vi "Configure.vi"(6 "CMD Prefix":string, 7 "CMDs":string[](array[string]), 8 "error in":errorcluster, 9 "JSON Settings Path":string, 10 "JSON Keys":string[](array[string]), 11 "Continuous Waveform Acq CFG in":refnum<class "Continuous Waveform Acq CFG.lvclass">) -> (0 "error out":errorcluster, 3 "Continuous Waveform Acq CFG out":refnum<class "Continuous Waveform Acq CFG.lvclass">)   [LabVIEW 2023, in "Continuous Waveform Acq CFG.lvclass"]
uses:
  Continuous Waveform Acq CFG.lvclass
  E:/git/HAL/Configuration Base/Configuration Base.lvclass
  E:/git/HAL/Scope VISA/Configuration/Scope VISA CFG.lvclass
  HAL/Scope VISA/Configuration/Scope VISA CFG.lvclass/Scope VISA CFG.ctl
  HAL/Configuration Base/Configuration Base.lvclass/Configuration Base.ctl
  <vilib>/JDP Science/JSONtext/Next JSON Value.vi
  <vilib>/JDP Science/JSONtext/String Subset.vi
  <vilib>/JDP Science/JSONtext/Parsing/Advance past next JSON Value (inlined COPY).vi
  <vilib>/JDP Science/JSONtext/Parsing/Advance past whitespace.vi
  <vilib>/JDP Science/JSONtext/Parsing/Advance past String.vi
  <vilib>/JDP Science/JSONtext/Parsing/Advance past Number.vi
  <vilib>/JDP Science/JSONtext/Parsing/Advance past Line Ending.vi
  <vilib>/JDP Science/JSONtext/Parsing/Parse Full Path or Item Name.vi
  <vilib>/JDP Science/JSONtext/Parsing/Advance past Array.vi
  <vilib>/JDP Science/JSONtext/Parsing/Advance past Object.vi
  <vilib>/JDP Science/JSONtext/support/Error Cluster From Code.vi
  <vilib>/JDP Science/JSONtext/Offset/Find Item Locations by Path.vi
  Continuous Waveform Acq CFG.lvclass/Continuous Waveform Acq CFG.ctl
  HAL/Scope VISA/Configuration/Scope VISA CFG.lvclass
  HAL/Configuration Base/Configuration Base.lvclass
  <vilib>/JDP Science/JSONtext/JSONtext.lvlib
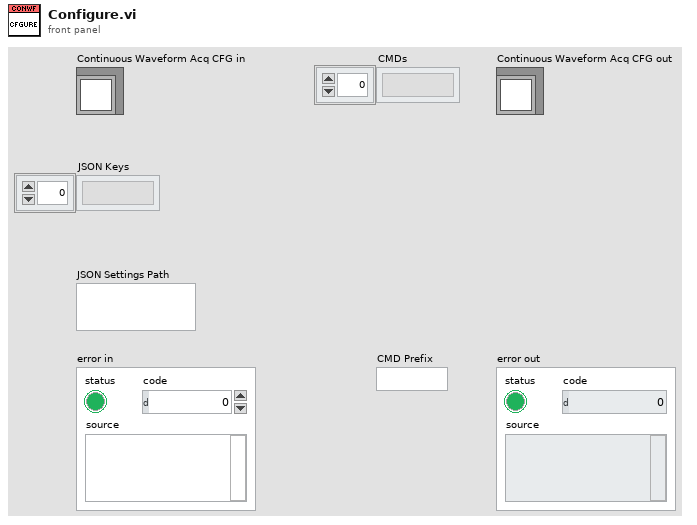
[diagram p1: front panel]
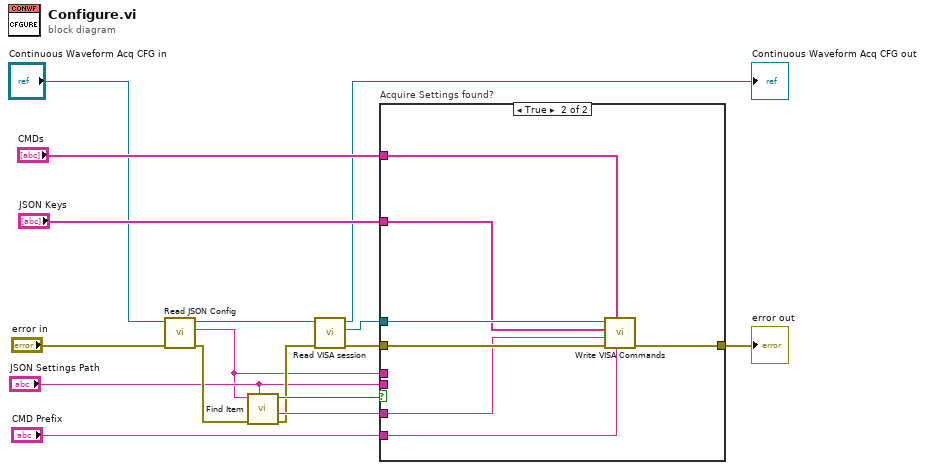
[diagram p0: block diagram]
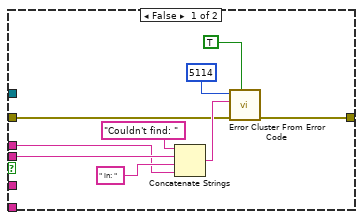
[diagram p2: hidden frame]
diagram:
  n1 = call "Read JSON Config.vi"("error in (no error)"="error in", "object in"="Continuous Waveform Acq CFG in") -> ("error out"=w4:errorcluster, "<JSON>Config"=w1:string, "object out"=w10:refnum<class "Continuous Waveform Acq CFG.lvclass">)  [unwired: 7 in]
  n2 = call <vilib>:"Find Item.vi"("$Path or Item Name"="JSON Settings Path", "error in (no error)"=w4, "JSON"=w1) -> ("error out"=w3:errorcluster, "<JSON>"=w13:string, "Found"=w11:bool)  [unwired: 5 in, 1 out]
  n3 = call "Read VISA session.vi"("error in (no error)"=w3, "Scope VISA CFG in"=w10) -> ("error out"=w12:errorcluster, "VISA session"=w7:refnum<visa-resource-name>, "Scope VISA CFG out"=→"Continuous Waveform Acq CFG out":refnum<class "Continuous Waveform Acq CFG.lvclass">)  [unwired: 7 in]
  n4 = case "Acquire Settings found?" shown="True" w11 {
    tunnel: [w25 w32] -> w5
    tunnel: w12 -> [w18 w31]
    tunnel: w7 -> [_ w30]
    tunnel: w13 -> [_ w29]
    tunnel: "CMD Prefix" -> [_ w28]
    tunnel: "CMDs" -> [_ w27]
    tunnel: "JSON Keys" -> [_ w26]
    tunnel: "JSON Settings Path" -> [w22 _]
    tunnel: w1 -> [w20 _]
    frame False {
      n5 = Concatenate Strings("Couldn't find: " ("string"), w22, " in: " ("string"), w20) -> (w19:string)
      n6 = call <vilib>:"Error Cluster From Error Code.vi"("show call chain? (False)"=TRUE, "error in (no error)"=w18, "error message (\"\")"=w19, "error code (0)"=5114) -> ("error out"=w25:errorcluster)  [unwired: 5 in]
    }
    frame True {
      n7 = call "Write VISA Commands.vi"("CMD Prefix"=w28, "CMDs"=w27, "error in"=w31, "<JSON> Object"=w29, "JSON Keys"=w26, "VISA Refnum in"=w30) -> ("error out"=w32:errorcluster)  [unwired: 4 in, 1 out]
    }
  }
  "error out" <- w5
